vi "sv_UFF58 Check Data Valid (Freq - Real) (NCh).vi"(5 "spectra":cluster{"f0":dbl, "df":dbl, "magnitude":dbl[]}[](array[cluster]) {"magnitude" format="%.2p"; "df" format="%.2p"; "f0" format="%.2p"}, 11 "error in (no error)":errorcluster) -> (6 "dup spectra":cluster{"f0":dbl, "df":dbl, "magnitude":dbl[]}[](array[cluster]) {"magnitude" format="%.2p"; "df" format="%.2p"; "f0" format="%.2p"}, 15 "error out":errorcluster)   [LabVIEW 2017, in "SoundVib_UFF58.lvlib"]
uses:
  <vilib>/addons/Sound and Vibration/svt_UFF58/SoundVib_UFF58.lvlib
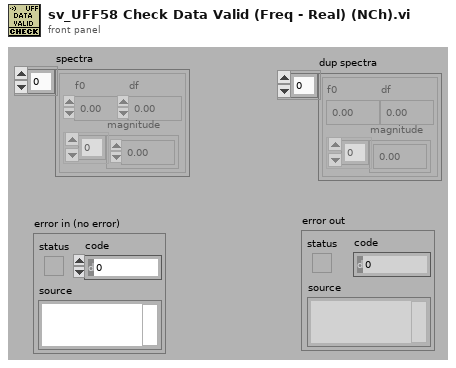
[diagram p1: front panel]
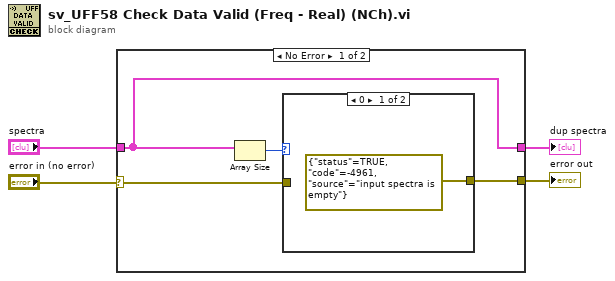
[diagram p0: block diagram]
diagram:
  n1 = case shown="No Error" "error in (no error)" {
    selector: "error in (no error)" -> [w6 w12]
    tunnel: "spectra" -> [w5 w11]
    tunnel: [w7 w12] -> w4
    tunnel: [w5 w11] -> w1
    frame No Error {
      n2 = Array Size(array=w5) -> (size(s)=w8:i32)
      n3 = case shown="0" w8 {
        tunnel: w6 -> [_ w10]
        tunnel: [errorcluster {"status"=TRUE, "code"=-4961, "source"="input spectra is empty"} ("error IO") w10] -> w7
        frame 0 {
        }
        frame 1, Default {
        }
      }
    }
    frame Error {
    }
  }
  "error out" <- w4
  "dup spectra" <- w1
